vi "Interface - Inheritance Parent Interfaces.vi"(7 "Msg Chain":string, 8 "error in (no error)":errorcluster {"code" format="Error %.0f"}, 10 "Interfaces":refnum<class "Interface Documenation.lvclass">[](array[class]), 11 "VIDoc Printer - Confluence In":refnum<class "VIDoc Printer - Confluence.lvclass">) -> (0 "error out":errorcluster {"code" format="Error %.0f"}, 3 "VIDoc Printer - Confluence Out":refnum<class "VIDoc Printer - Confluence.lvclass">)   [LabVIEW 2023, in "VIDoc Printer - Confluence.lvlib" / "VIDoc Printer - Confluence.lvclass"]
uses:
  VIDoc Printer - Confluence.lvclass
  C:/projects/DMC/Tooling/Git-Action-Service/Source/Documentation Generation/Printers/Printer/VIDoc Printer.lvclass
  Parsing/Interface Documenation/Interface Documenation.lvclass
  Parsing/Interface Documenation/Interface Documenation.lvclass/Interface Documenation.ctl
  Confluence Formatting/Types/Format Combo Box.ctl
  Settings/Printer Settings/Detail Level Enum.ctl
  Parsing/Interface Documenation/Get Parent Interfaces.vi
  Parsing/Interface Documenation/Get Name.vi
  VIDoc Printer - Confluence.lvclass/VIDoc Printer - Confluence.ctl
  Printer/VIDoc Printer.lvclass
  UI Interaction/UI Interaction.lvclass
  Confluence Formatting/Confluence Formatting.lvlib
  Settings/Printer Settings/Printer Settings.lvclass
  C:/projects/DMC/Tooling/Git-Action-Service/Source/Documentation Generation/Printers/Confluence Printer/VIDoc Printer - Confluence.lvclass
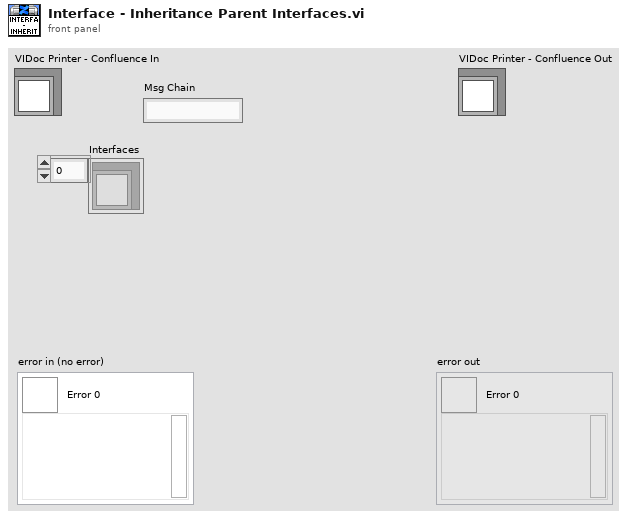
[diagram p1: front panel]
types:
  T1 = typedef "VIDoc Printer.lvlib/Printer Settings.lvclass/Detail Level Enum.ctl" = enum16{"None", "Minimal", "Standard", "Full"}
  T2 = typedef "Confluence Formatting.lvlib/Format Combo Box.ctl" = string
  T3 = typedef "VIDoc Parsing.lvlib/Base Class Info Cluster.ctl" = cluster{"Name":string, "Icon":T4, "Version":cluster{"Major":u16, "Minor":u16, "Fix":u16, "Build":u16}, "Description":string, "Friends":string[], "ChildRefsRestricted":bool, "TransferMustOverrides":bool, "Path":path, "Qualified Name":string, "Class Scope":enum32{"invalid scope", "public", "private", "protected", "community"}}
  T4 = typedef "imagedata.ctl" = cluster{"image type":i32, "image depth":i32, "image":u8[], "mask":u8[], "colors":u32[], "Rectangle":cluster{"left":i16, "top":i16, "right":i16, "bottom":i16}}
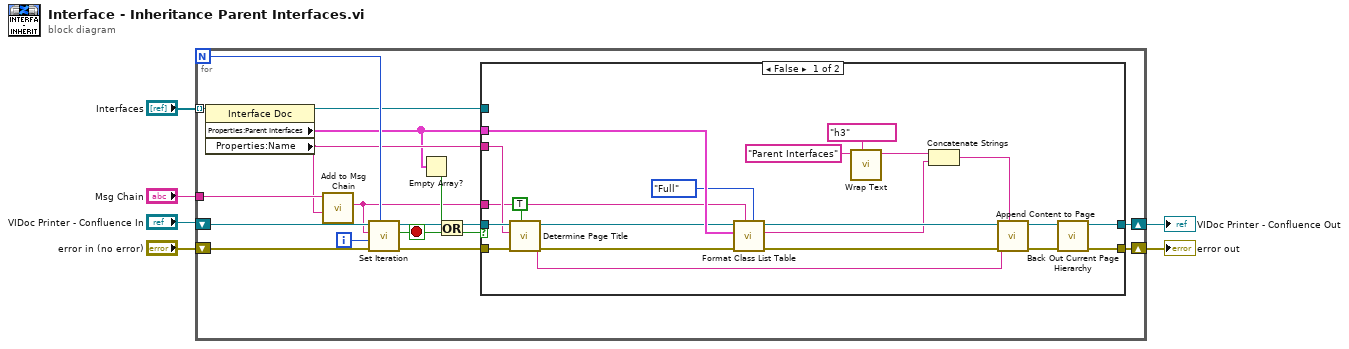
[diagram p0: block diagram]
diagram:
  n1 = for {
    N -> [w16]
    shift-right: [w21] -> w6
    shift-left: "error in (no error)" -> [w19]
    shift-right: [w22] -> w5
    shift-left: "VIDoc Printer - Confluence In" -> [w20]
    tunnel: "Interfaces" -> [w23] mode=indexing
    tunnel: "Msg Chain" -> [w14]
    i -> [w15]
    stop <- w12 stop-if-true
    n2 = property class="Interface Doc"(reference=w23) -> (reference out=w11:refnum<class "Interface Documenation.lvclass">, "Properties:Parent Interfaces"=w10:T3[], "Properties:Name"=w13:string)  [unwired: 1 in, 1 out]
    n3 = call "Add to Msg Chain.vi"("New"=w13, "Msg Chain in"=w14) -> ("Msg Chain out"=w7:string)  [unwired: 9 in]
    n4 = call "Set Iteration.vi"("Progress Max"=w16, "error in (no error)"=w19, "Progress Value"=w15, "Message (No Message Update)"=w7, "VIDoc Printer In"=w20) -> ("error out"=w17:errorcluster, "Abort?"=w12:bool, "VIDoc Printer Out"=w18:refnum<class "VIDoc Printer - Confluence.lvclass">)  [unwired: 4 in]
    n5 = Empty Array?(array=w10) -> (empty?=w8:bool)
    n6 = Or(x=w8, y=w12) -> (x .or. y?=w9:bool)
    n7 = case shown="False" w9 {
      tunnel: [w25 w45] -> w22
      tunnel: [w27 w46] -> w21
      tunnel: w10 -> [w36 _]
      tunnel: w18 -> [w41 w45]
      tunnel: w17 -> [w40 w46]
      tunnel: w13 -> [w39 _]
      tunnel: w11 -> [_ _]
      tunnel: w7 -> [w29 _]
      frame False {
        n8 = call "Determine Page Title.vi"("Update Current Page (F)"=TRUE, "error in (no error)"=w40, "Name"=w39, "VIDoc Printer - Confluence In"=w41) -> ("error out"=w35:errorcluster, "Page Title"=w44:string, "VIDoc Printer - Confluence Out"=w33:refnum<class "VIDoc Printer - Confluence.lvclass">)  [unwired: 4 in, 1 out]
        n9 = call "Format Class List Table.vi"("Detail Level"=Detail_Level_Enum."Full", "Msg Chain in"=w29, "error in (no error)"=w35, "Class Info Array"=w36, "VIDoc Printer - Confluence In"=w33) -> ("error out"=w34:errorcluster, "Table Text"=w30:string, "VIDoc Printer - Confluence Out"=w32:refnum<class "VIDoc Printer - Confluence.lvclass">)  [unwired: 4 in]
        n10 = call "Wrap Text.vi"("Formatting"=T2 "h3", "String"="Parent Interfaces") -> ("Wrapped String"=w37:string)  [unwired: 8 in, 1 out]
        n11 = Concatenate Strings(w37, w30) -> (w31:string)
        n12 = call "Append Content to Page.vi"("Page Content"=w31, "error in (no error)"=w34, "Page Title"=w44, "VIDoc Printer - Confluence In"=w32) -> ("error out"=w43:errorcluster, "VIDoc Printer - Confluence Out"=w26:refnum<class "VIDoc Printer - Confluence.lvclass">)  [unwired: 6 in]
        n13 = call "Back Out Current Page Hierarchy.vi"("error in (no error)"=w43, "VIDoc Printer - Confluence In"=w26) -> ("error out"=w27:errorcluster, "VIDoc Printer - Confluence Out"=w25:refnum<class "VIDoc Printer - Confluence.lvclass">)  [unwired: 8 in]
      }
      frame True {
      }
    }
  }
  "error out" <- w6
  "VIDoc Printer - Confluence Out" <- w5
